vi "PathPlanner_EventMarkerExecute.vi"(9 "EventMarkers":T1[](array[typedef]) {"lastRobotPos"."Y" format="%14.3f"; "lastRobotPos"."X" format="%14.3f"; "markerPos"."Y" format="%14.3f"; "markerPos"."X" format="%14.3f"}, 11 "Event Name":string="Shoot 1") -> (0 "Event End":bool, 2 "Event Request":bool, 3 "Timers":dbl[](array[numeric]))   [LabVIEW 2023]
uses:
  <vilib>/Rock Robotics/WPI/ThirdParty/MJansen/PathPlanner/TypeDef/PathPlannerEventMarker.ctl
  <vilib>/Rock Robotics/WPI/ThirdParty/JAS_Junk/TrajLib/TypeDef/TRANSLATION2D.ctl
  <vilib>/Rock Robotics/WPI/ThirdParty/MJansen/PathPlanner/TypeDef/PathPlannerCommandUtil.ctl
  <vilib>/Rock Robotics/WPI/ThirdParty/MJansen/PathPlanner/ENum/PathPlanner_CommandUtilType_ENUM.ctl
  <vilib>/Rock Robotics/WPI/ThirdParty/JAS_Junk/TrajLib/VI/BoolCmd_Recv_Internal.vi
  <vilib>/Rock Robotics/WPI/ThirdParty/JAS_Junk/TrajLib/VI/BoolCmd_Send_Internal.vi
  <vilib>/Rock Robotics/WPI/ThirdParty/JAS_Junk/TrajLib/VI/BoolCmd_ObtainQueue.vi
  <vilib>/Utility/semaphor.llb/Obtain Semaphore Reference.vi
  <vilib>/Rock Robotics/WPI/ThirdParty/JAS_Junk/TrajLib/Timer_Reset.vi
  <vilib>/Rock Robotics/WPI/ThirdParty/MJansen/PathPlanner/PathPlanner24.lvlib
  <vilib>/Rock Robotics/WPI/ThirdParty/JAS_Junk/TrajLib/Trajectory_Library.lvlib
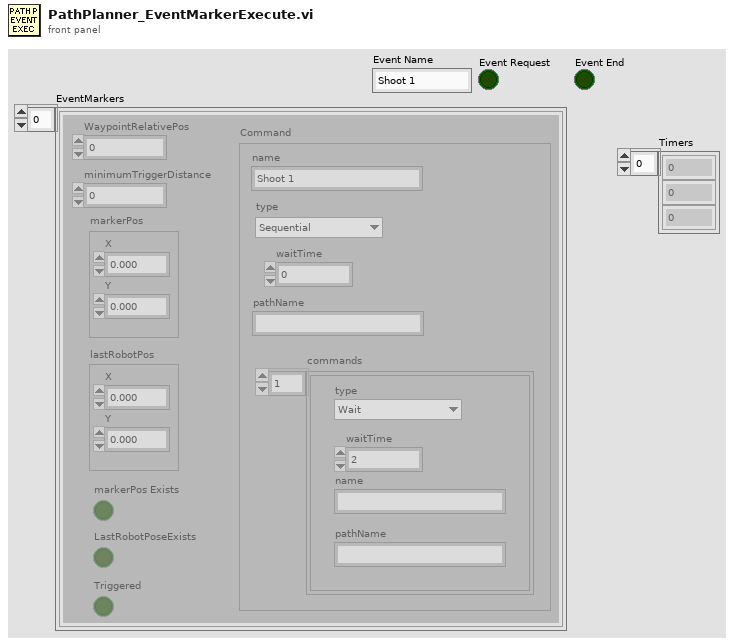
[diagram p1: front panel]
types:
  T1 = typedef "PathPlanner24.lvlib/PathPlannerEventMarker.ctl" = cluster{"WaypointRelativePos":dbl, "minimumTriggerDistance":dbl, "markerPos":T2, "lastRobotPos":T2, "Command":T3, "markerPos Exists":bool, "LastRobotPoseExists":bool, "Triggered":bool}
  T2 = typedef "Trajectory_Library.lvlib/TRANSLATION2D.ctl" = cluster{"X":dbl, "Y":dbl}
  T3 = typedef "PathPlanner24.lvlib/PathPlannerCommandUtil.ctl" = cluster{"waitTime":dbl, "name":string, "pathName":string, "commands":cluster{"type":T4, "waitTime":dbl, "name":string, "pathName":string}[], "type":T4}
  T4 = typedef "PathPlanner24.lvlib/PathPlanner_CommandUtilType_ENUM.ctl" = enum16{"Unknown", "Wait", "Named", "Path", "Sequential", "Parallel", "Race", "Deadline"}
  T5 = cluster{"type":T4, "waitTime":dbl, "name":string, "pathName":string}[]
  T6 = typedef "Trajectory_Library.lvlib/TIMER.ctl" = cluster{"StartTime":dbl, "Accumulated TIme":dbl, "Running":bool, "semaphore":T7}
  T7 = typedef "Semaphore RefNum" = refnum<k1>
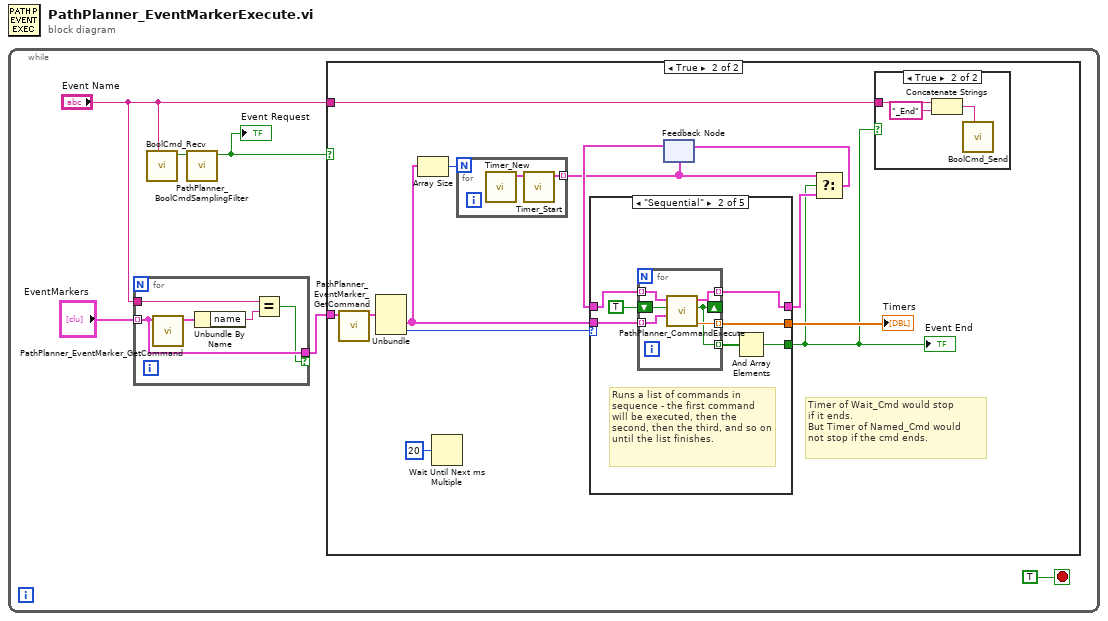
[diagram p0: block diagram]
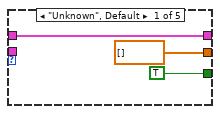
[diagram p4: hidden frame]
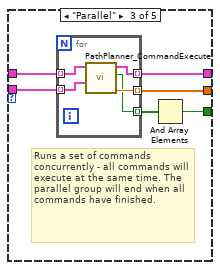
[diagram p5: hidden frame]
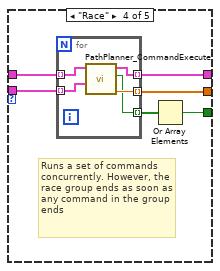
[diagram p6: hidden frame]
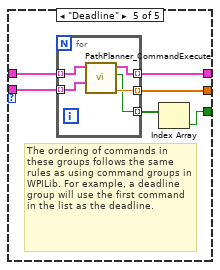
[diagram p7: hidden frame]
diagram:
  n1 = while {
    stop <- TRUE stop-if-true
    n2 = for {
      tunnel: "EventMarkers" -> [w75] mode=indexing
      tunnel: "Event Name" -> [w77]
      tunnel: [w75] -> w6 if=w74
      n3 = call <vilib>:"PathPlanner_EventMarker_GetCommand.vi"("in EventMarker"=w75) -> ("Command"=w78:T3)  [unwired: 10 in]
      n4 = Unbundle By Name(w78) -> ("name"=w76:string)
      n5 = Equal?(x=w77, y=w76) -> (x = y?=w74:bool)
    }
    n6 = call <vilib>:"BoolCmd_Recv.vi"("Command Name"="Event Name") -> ("New Request"=w4:bool)  [unwired: 9 in, 1 out]
    n7 = call "PathPlanner_BoolCmdSamplingFilter.vi"("Input"=w4) -> ("Output"=w2:bool)  [unwired: 10 in]
    "Event Request" <- w2
    n8 = case shown="True" w2 {
      tunnel: w6 -> [_ w19]
      tunnel: "Event Name" -> [_ w8]
      frame False {
      }
      frame True {
        # "Timer of Wait_Cmd would stop \nif it ends.\nBut Timer of Named_Cmd would \nnot stop if the cmd ends."
        n9 = call <vilib>:"PathPlanner_EventMarker_GetCommand.vi"("in EventMarker"=w19) -> ("Command"=w18:T3)  [unwired: 10 in]
        n10 = Unbundle(w18) -> ("commands"=w15:T5, "type"=w17:T4)  [unwired: 3 out]
        n11 = Array Size(array=w15) -> (size(s)=w16:i32)
        n12 = Wait Until Next ms Multiple(millisecond multiple=u32 20 ("milliseconds to wait")) -> ()  [unwired: 1 out]
        n13 = for {
          N: w16 -> [_]
          tunnel: [w23] -> w10 mode=indexing
          n14 = call <vilib>:"Timer_New.vi"() -> ("TIMER"=w24:T6)  [unwired: 11 in]
          n15 = call <vilib>:"Timer_Start.vi"("in Timer"=w24) -> ("out Timer"=w23:T6)  [unwired: 10 in]
        }
        n16 = feedback #1(w10) -> (w12:T6[])
        n17 = case shown="\"Sequential\"" w17 {
          tunnel: w15 -> [_ w34 w46 w57 w68]
          tunnel: [dbl[] [] w32 w45 w56 w67] -> w14
          tunnel: [w25 w31 w44 w55 w63] -> w11
          tunnel: [TRUE w29 w42 w53 w65] -> w7
          tunnel: w12 -> [w25 w28 w41 w52 w64]
          frame "Unknown", Default {
          }
          frame "Sequential" {
            # "Runs a list of commands in sequence - the first command will be executed, then the second, then the third, and so on until the list finishes."
            n18 = for {
              tunnel: w34 -> [w40] mode=indexing
              shift-right: [w35] -> _
              shift-left: TRUE ("Expired") -> [w39]
              tunnel: [w38] -> w31 mode=indexing
              tunnel: w28 -> [w37] mode=indexing
              tunnel: [w36] -> w32 mode=indexing
              tunnel: [w35] -> w30 mode=indexing
              n19 = call "PathPlanner_CommandExecute.vi"("command"=w40, "Execute"=w39, "in Timer"=w37) -> ("CurrentTImer"=w36:dbl, "Expired"=w35:bool, "out Timer"=w38:T6)  [unwired: 6 in]
            }
            n20 = And Array Elements(Boolean array=w30) -> (logical AND=w29:bool)
          }
          frame "Parallel" {
            # "Runs a set of commands concurrently - all commands will execute at the same time. The parallel group will end when all commands have finished."
            n21 = for {
              tunnel: w46 -> [w51] mode=indexing
              tunnel: [w50] -> w44 mode=indexing
              tunnel: w41 -> [w49] mode=indexing
              tunnel: [w48] -> w45 mode=indexing
              tunnel: [w47] -> w43 mode=indexing
              n22 = call "PathPlanner_CommandExecute.vi"("command"=w51, "in Timer"=w49) -> ("CurrentTImer"=w48:dbl, "Expired"=w47:bool, "out Timer"=w50:T6)  [unwired: 7 in]
            }
            n23 = And Array Elements(Boolean array=w43) -> (logical AND=w42:bool)
          }
          frame "Race" {
            # "Runs a set of commands concurrently. However, the race group ends as soon as any command in the group ends"
            n24 = for {
              tunnel: w57 -> [w62] mode=indexing
              tunnel: [w61] -> w55 mode=indexing
              tunnel: w52 -> [w60] mode=indexing
              tunnel: [w59] -> w56 mode=indexing
              tunnel: [w58] -> w54 mode=indexing
              n25 = call "PathPlanner_CommandExecute.vi"("command"=w62, "in Timer"=w60) -> ("CurrentTImer"=w59:dbl, "Expired"=w58:bool, "out Timer"=w61:T6)  [unwired: 7 in]
            }
            n26 = Or Array Elements(Boolean array=w54) -> (logical OR=w53:bool)
          }
          frame "Deadline" {
            # "The ordering of commands in these groups follows the same rules as using command groups in WPILib. For example, a deadline group will use the first command in the list as the deadline."
            n27 = for {
              tunnel: w68 -> [w73] mode=indexing
              tunnel: [w72] -> w63 mode=indexing
              tunnel: w64 -> [w71] mode=indexing
              tunnel: [w70] -> w67 mode=indexing
              tunnel: [w69] -> w66 mode=indexing
              n28 = call "PathPlanner_CommandExecute.vi"("command"=w73, "in Timer"=w71) -> ("CurrentTImer"=w70:dbl, "Expired"=w69:bool, "out Timer"=w72:T6)  [unwired: 7 in]
            }
            n29 = Index Array(array=w66) -> (element=w65:bool)  [unwired: 1 in]
          }
        }
        "Timers" <- w14
        "Event End" <- w7
        n30 = Select(t=w10, s=w7, f=w11) -> (s? t:f=w9:T6[])
        n31 = feedback-in #1(w9) -> ()
        n32 = case shown="True" w7 {
          tunnel: w8 -> [_ w21]
          frame False {
          }
          frame True {
            n33 = Concatenate Strings(w21, "_End" ("string")) -> (w20:string)
            n34 = call <vilib>:"BoolCmd_Send.vi"("Command Name"=w20) -> ()  [unwired: 10 in, 1 out]
          }
        }
      }
    }
  }
